vi "Get LakeShore 340 Formated Parameters.vi"(0 "VISA Resource Name":refnum<visa-resource-name>, 1 "Initial String":string, 5 "error in (no error)":errorcluster) -> (7 "Parameters":string, 13 "Data titles":string[](array[string])=["LS340_T (K)", "LS340_R (Ohm)"], 14 "VISA Resource Name Out":refnum<visa-resource-name>, 19 "error out":errorcluster)   [LabVIEW 2015]
uses:
  GPIB/VISA  Send Receive.vi
panel:
  in  "Offset":i32
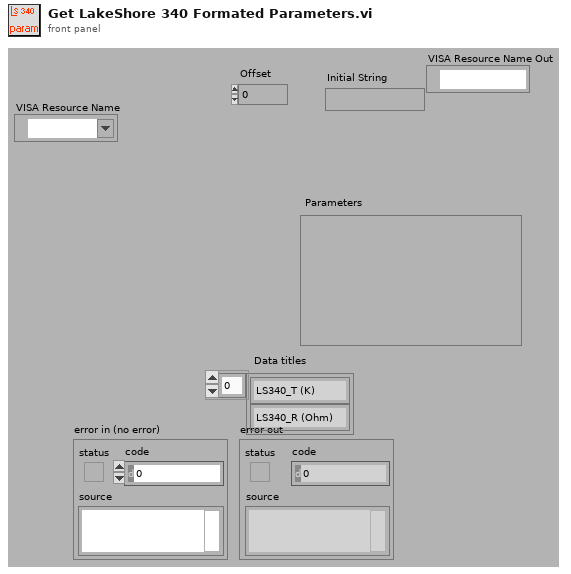
[diagram p1: front panel]
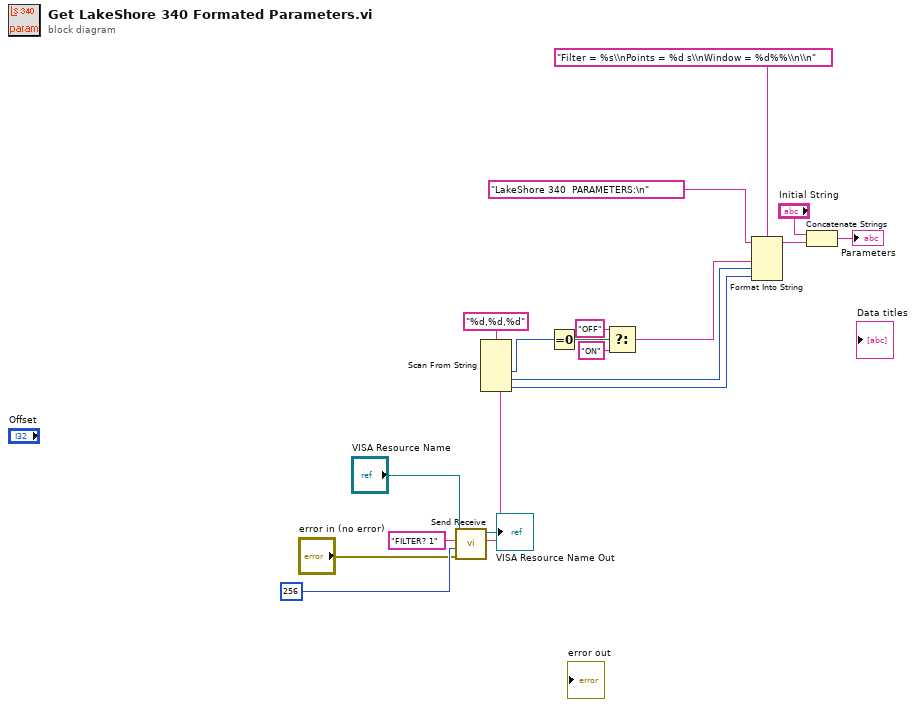
[diagram p0: block diagram]
diagram:
  n1 = call-poly "Send Receive.vi"("error in (no error)"="error in (no error)", "Receive count"=256, "data string in"="FILTER? 1", "VISA Resource Name"="VISA Resource Name") -> ("data string out"=w16:string, "VISA Resource Name Out"=→"VISA Resource Name Out":refnum<visa-resource-name>)  [unwired: 5 in, 1 out]
  n2 = Scan From String(format string="%d,%d,%d", input string=w16) -> (output 1=w12:i32, output 2=w5:i32, output 3=w4:i32)  [unwired: 2 in, 6 out]
  n3 = Equal To 0?(x=w12) -> (x = 0?=w15:bool)
  n4 = Select(t="OFF", s=w15, f="ON") -> (s? t:f=w6:string)
  n5 = Format Into String(format string="Filter = %s\\nPoints = %d s\\nWindow = %d%%\\n\\n", initial string="LakeShore 340  PARAMETERS:\n", w6, w5, w4) -> (resulting string=w10:string)  [unwired: 1 in, 1 out]
  n6 = Concatenate Strings("Initial String", w10) -> (→"Parameters":string)
